vi "Evaluate Expression.vi"(8 "error in (no error)":errorcluster, 10 "Expression":string, 11 "Session Handle in":refnum<data-value>) -> (0 "error out":errorcluster, 2 "Python Object Refnum":T1, 3 "Session Handle out":refnum<data-value>)   [LabVIEW 2020, in "G-Embedded-Python-Interpreter-Toolkit.lvlib"]
uses:
  G-Embedded-Python-Interpreter-Toolkit.lvlib
  Python Object Reference.ctl
  Python Object Type.ctl
  bin/gepit.cp310.32.dll
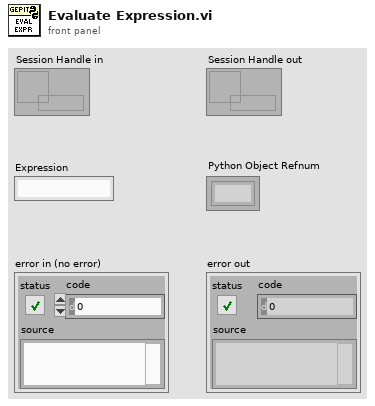
[diagram p1: front panel]
types:
  T1 = typedef "G-Embedded-Python-Interpreter-Toolkit.lvlib/Python Object Reference.ctl" = refnum<k1>
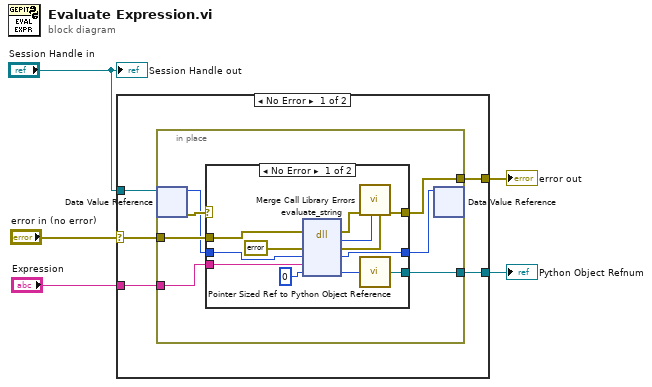
[diagram p0: block diagram]
diagram:
  n1 = case shown="No Error" "error in (no error)" {
    selector: "error in (no error)" -> [w9 w32]
    tunnel: "Session Handle in" -> [w10 _]
    tunnel: [w8 w32] -> w4
    tunnel: [w7 _] -> w1
    tunnel: "Expression" -> [w6 _]
    frame No Error {
      n2 = in-place {
        in-place-border: w9 -> [w16]
        in-place-border: [w13] -> w8
        in-place-border: [w12] -> w7
        in-place-border: w6 -> [w11]
        n3 = in-place-dvr #1(w10) -> (w15:u64, w17:errorcluster)
        n4 = case shown="No Error" w17 {
          selector: w17 -> [_ w30]
          tunnel: w16 -> [w25 _]
          tunnel: w15 -> [w24 w31]
          tunnel: [w23 w31] -> w14
          tunnel: [w22 w30] -> w13
          tunnel: [w18 _] -> w12
          tunnel: w11 -> [w20 _]
          frame No Error {
            n5 = dll-call lib="C:/serenial/libraries/g-embedded-python-interpreter-toolkit/LabVIEW/bin/gepit.cp310.32.dll" fn="evaluate_string"(error in=w25, "Error"=errorcluster {"status"=FALSE, "code"=0, "source"=""} ("error constant"), "Session"=w24, "Expression"=w20, "Py Object"=u64 0) -> (error out=w28:errorcluster, "return type"=w27:i32, "Error"=w26:errorcluster, "Session"=w23:u64, "Py Object"=w21:u64)  [unwired: 3 in, 1 out]
            n6 = call "Merge Call Library Errors.vi"("Call Library Error"=w26, "Return Value"=w27, "error in"=w28) -> ("error out"=w22:errorcluster)  [unwired: 8 in]
            n7 = call "Pointer Sized Ref to Python Object Reference.vi"("Py Object in"=w21) -> ("Refnum out"=w18:T1)
          }
          frame Error {
          }
        }
        n8 = in-place-dvr #1(w14) -> ()  [unwired: 2 out]
      }
    }
    frame Error {
    }
  }
  "error out" <- w4
  "Python Object Refnum" <- w1
  "Session Handle out" <- "Session Handle in"
